vi "G_Boat Speed.vi"() -> ()   [LabVIEW 2012]
panel:
  out "Boat Speed":dbl
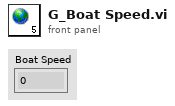
[diagram p1: front panel]
diagram:
